vi "Divide.vi"(8 "error in (no error)":errorcluster, 10 "Divider":dbl, 11 "Data1D in":refnum<class "Data1D.lvclass">) -> (0 "error out":errorcluster, 3 "Data1D out":refnum<class "Data1D.lvclass">)   [LabVIEW 2014, in "Data1D.lvclass"]
uses:
  Data1D.lvclass
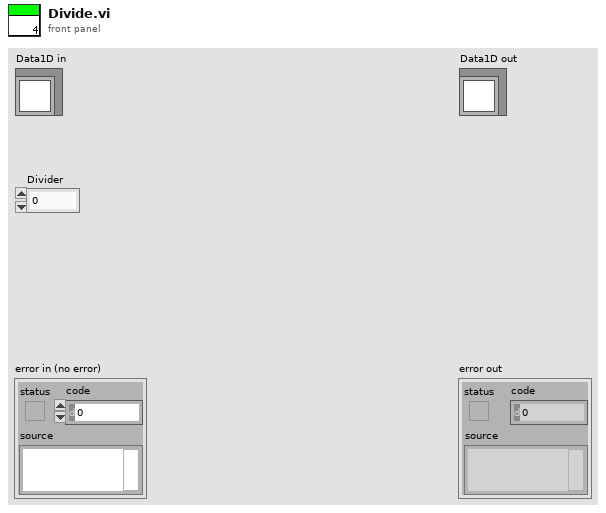
[diagram p1: front panel]
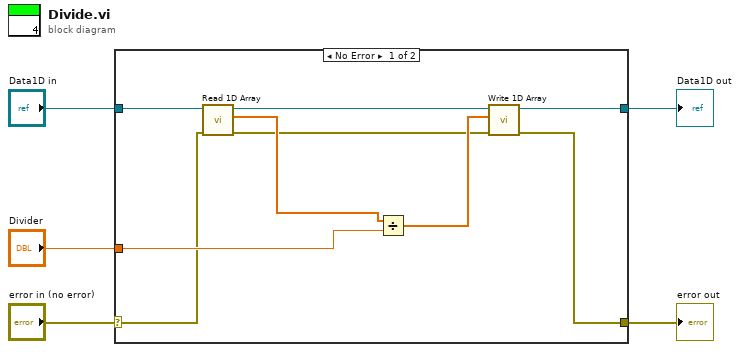
[diagram p0: block diagram]
diagram:
  n1 = case shown="No Error" "error in (no error)" {
    selector: "error in (no error)" -> [w13 w16]
    tunnel: [w6 w16] -> w4
    tunnel: [w10 w15] -> w2
    tunnel: "Data1D in" -> [w11 w15]
    tunnel: "Divider" -> [w14 _]
    frame No Error {
      n2 = call "Read 1D Array.vi"("error in (no error)"=w13, "Data1D in"=w11) -> ("error out"=w7:errorcluster, "1D Array"=w12:dbl[], "Data1D out"=w9:refnum<class "Data1D.lvclass">)  [unwired: 7 in]
      n3 = Divide(x=w12, y=w14) -> (x/y=w8:dbl[])
      n4 = call "Write 1D Array.vi"("error in (no error)"=w7, "1D Array"=w8, "Data1D in"=w9) -> ("error out"=w6:errorcluster, "Data1D out"=w10:refnum<class "Data1D.lvclass">)  [unwired: 7 in]
    }
    frame Error {
    }
  }
  "error out" <- w4
  "Data1D out" <- w2
